vi "反应性主程序.vi"() -> ()   [LabVIEW 2020]
doc: "该范例演示了通过VI查看其它VI的方法，还可运行和中止查看的VI。\n对于要中止的VI，应设置为可中止。对于无法中止的VI，可查看相关范例。"
uses:
  <vilib>/Utility/error.llb/DialogType.ctl
  GlobalVariable.vi
  TCPModbus_MasterClient/MB Ethernet Master Query Write Multiple Registers (poly).vi
  TCPModbus_MasterClient/MB Ethernet Master Query Read Input Registers (poly).vi
  <vilib>/Analysis/polynomials.llb/Scalar Polynomial Evaluation (DBL).vi
  <vilib>/Analysis/NI_AALPro.lvlib
panel:
  out "上段":bool
  out "下段":bool
  in  "修正因子文件状态":bool
  out "退出":bool
  in  "Calculate Square":bool
  in  "Measure Square":bool
  in  "Physics Parameters Square":bool
  in  "Open Square":bool
  in  "Home Square":bool
  out "时间":string
  out "日期":string
  in  "MainPanel":enum32{"logo"}(tab)
  out "P2_8":dbl
  out "P2_7":dbl
  out "P2_6":dbl
  out "P2_5":dbl
  out "P2_4":dbl
  out "P2_3":dbl
  out "P2_2":dbl
  out "P2_1":dbl
  out "累计时差":dbl format="%#_2g"
  out "程序历时":dbl format="%#_2g"
  out "电脑历时":dbl format="%#_2g"
  out "脉冲3":dbl(knob) caption="Gauge" scale=1.0..1000000.0 scale format="%#_6p"
  out "脉冲2":dbl(knob) caption="Gauge" scale=1.0..1000000.0 scale format="%#_6p"
  out "电流 2":dbl(slide)=1.0 scale=1e-13..0.0001 scale format="%#_2e"
  out "电流 1":dbl(slide)=1.0 scale=1e-13..0.0001 scale format="%#_2e"
  out "电压8":dbl(knob) caption="Gauge" scale=1.0..5.0
  out "电压7":dbl(knob) caption="Gauge" scale=1.0..5.0
  out "电压6":dbl(knob) caption="Gauge" scale=1.0..5.0
  out "电压5":dbl(knob) caption="Gauge" scale=1.0..5.0
  out "电压4":dbl(knob) caption="Gauge" scale=1.0..5.0
  out "电压3":dbl(knob) caption="Gauge" scale=1.0..5.0
  out "电压2":dbl(knob) caption="Gauge" scale=1.0..5.0
  out "脉冲1":dbl(knob) caption="Gauge" scale=1.0..1000000.0 scale format="%#_6p"
  out "电压1":dbl(knob) caption="Gauge" scale=1.0..5.0
  in  "校准时间":bool
  in  "更新物理参数":bool
  in  "离线数据源":bool
  # "iRho-100型反应性仪"
  # "Network"
  # "Current1"
  # "Current2"
  # "Voltage Output"
  # "Voltage Input"
  # "AC220V/50Hz"
  # "Ground"
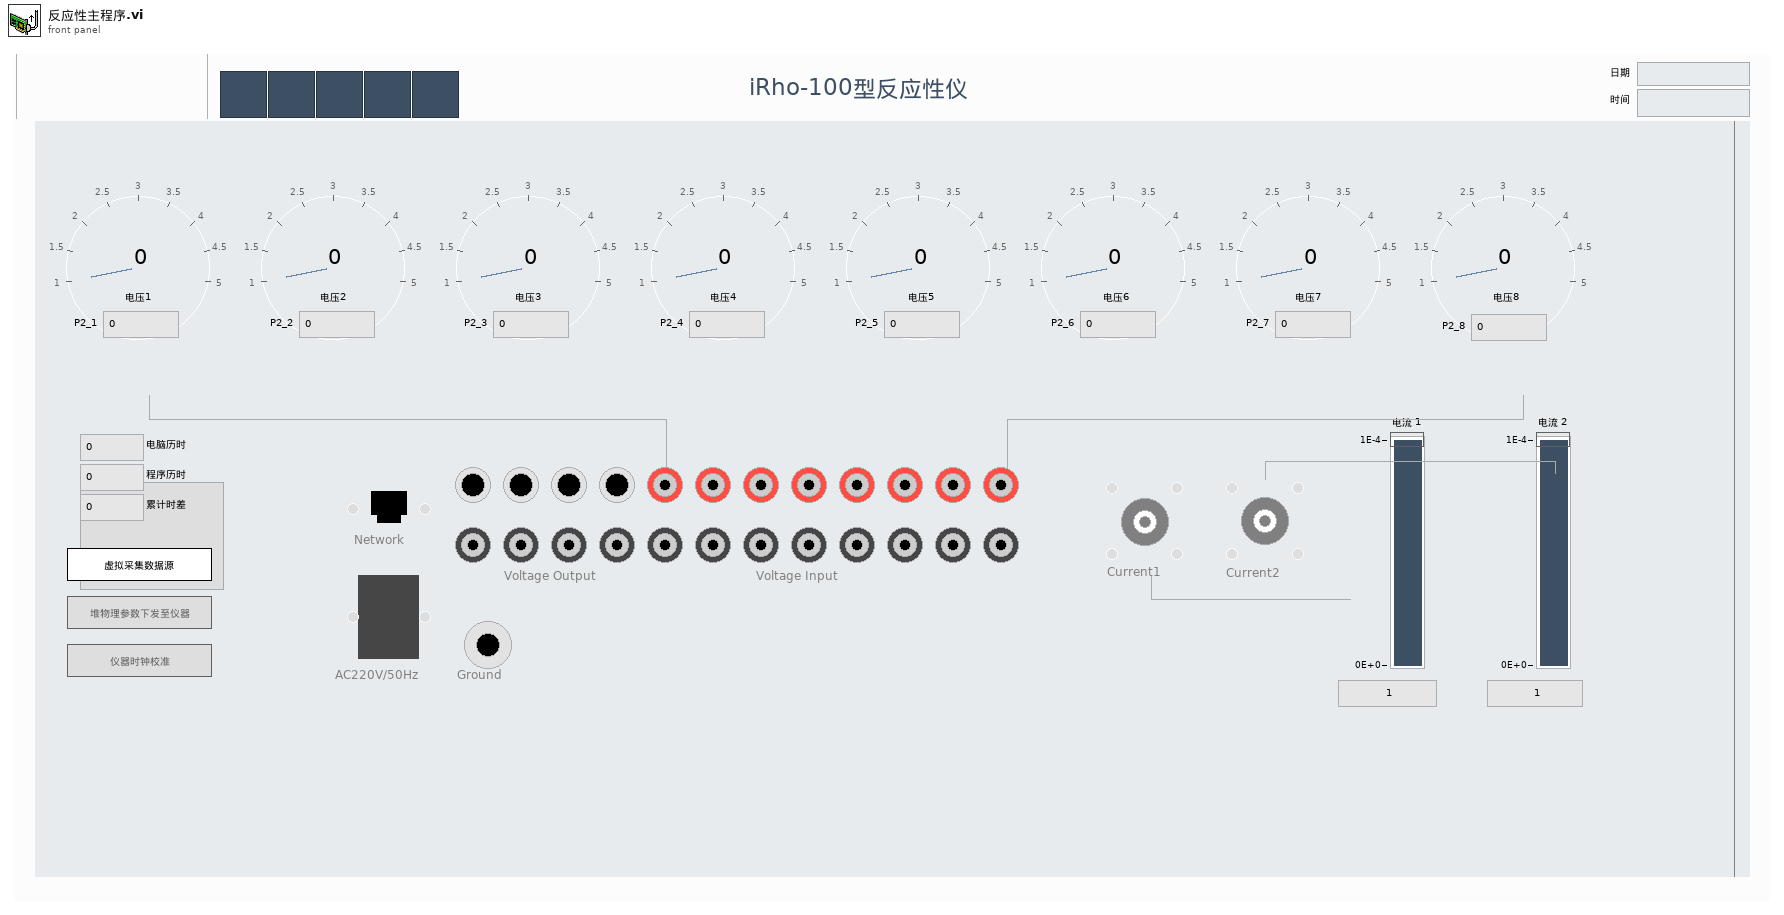
[diagram p1: front panel]
types:
  T1 = typedef "DialogType.ctl" = u16
  T2 = enum32{"Invalid", "Standard", "Closed", "Hidden", "Minimized", "Maximized"}
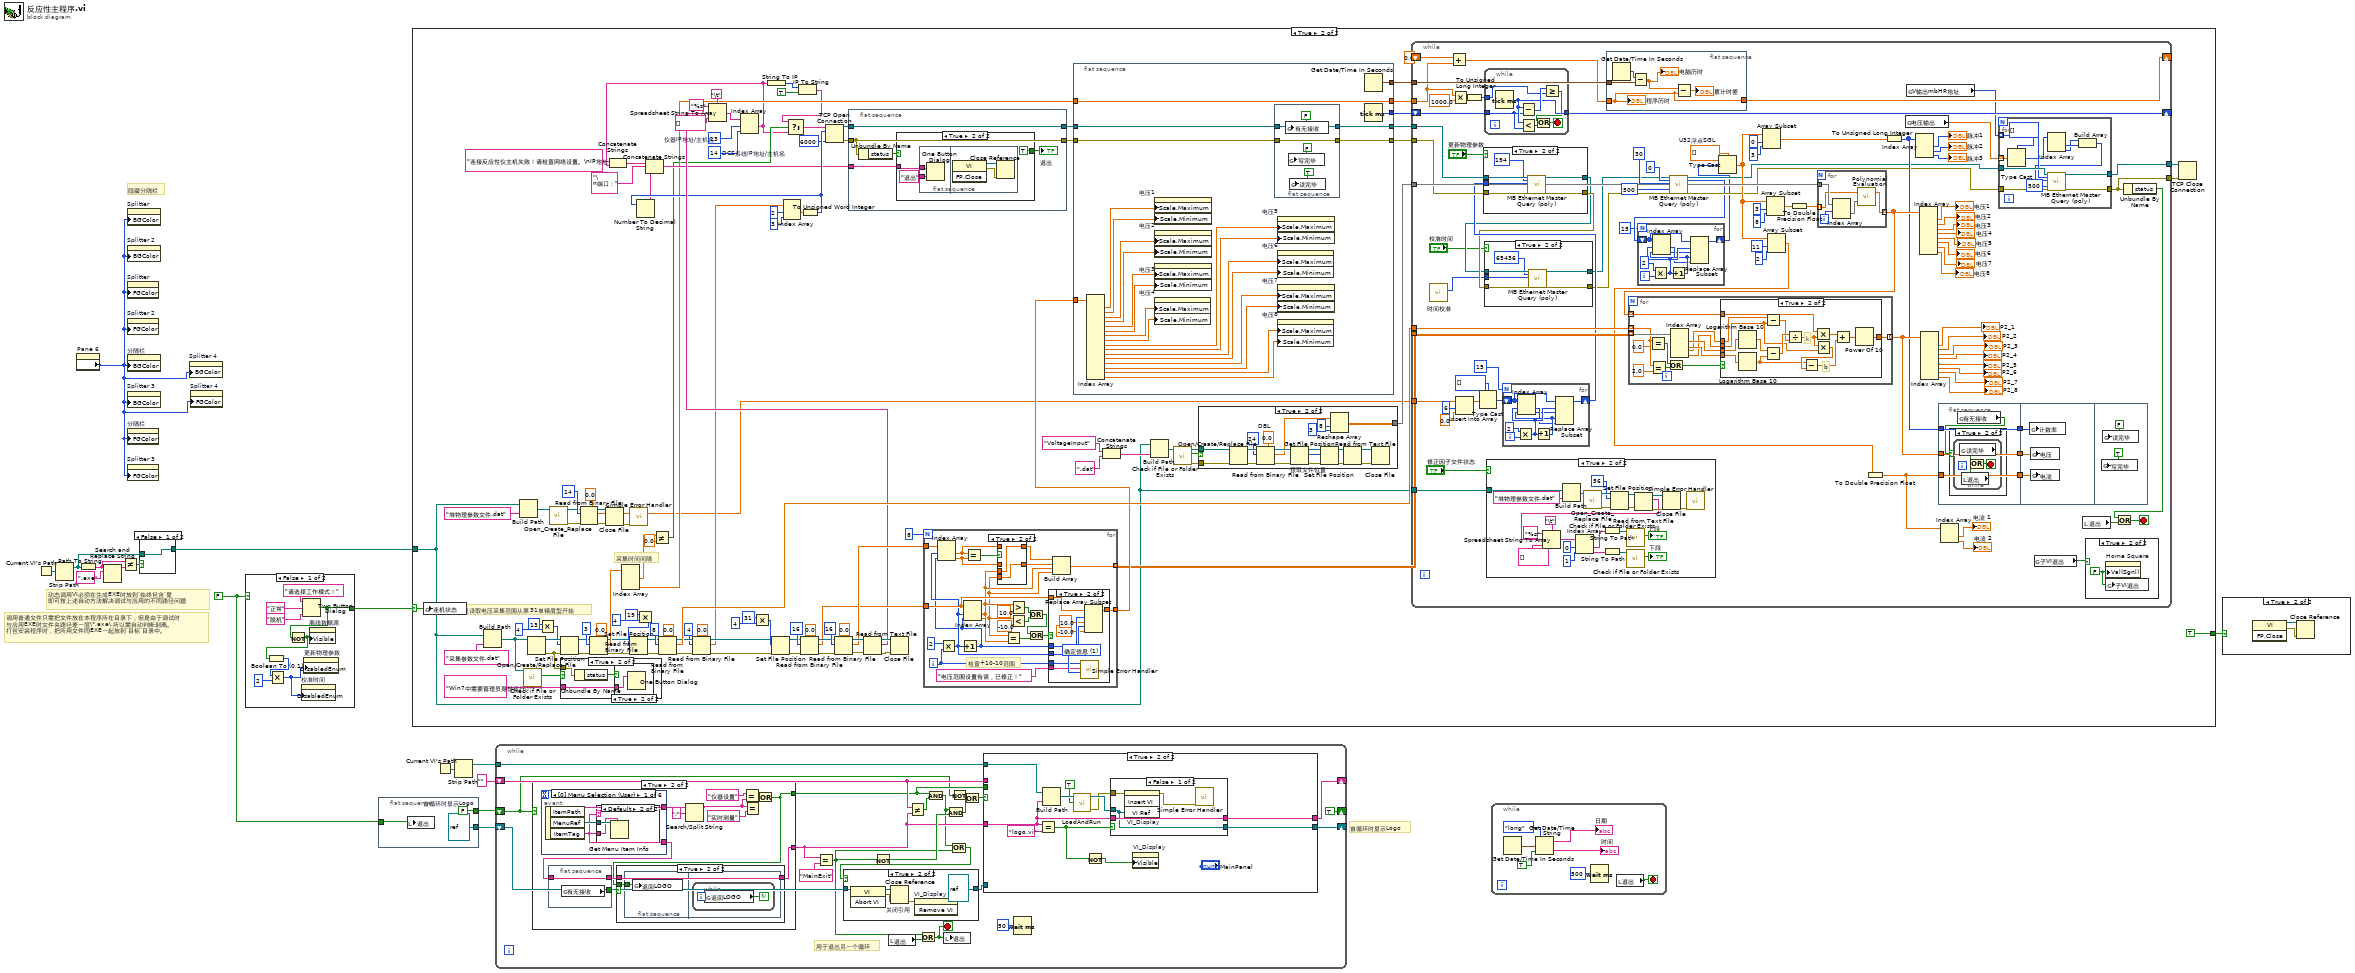
[diagram p0: block diagram]
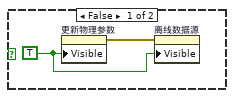
[diagram p2: hidden frame]
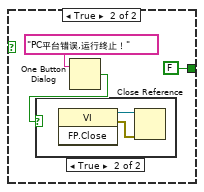
[diagram p3: hidden frame]
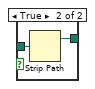
[diagram p5: hidden frame]
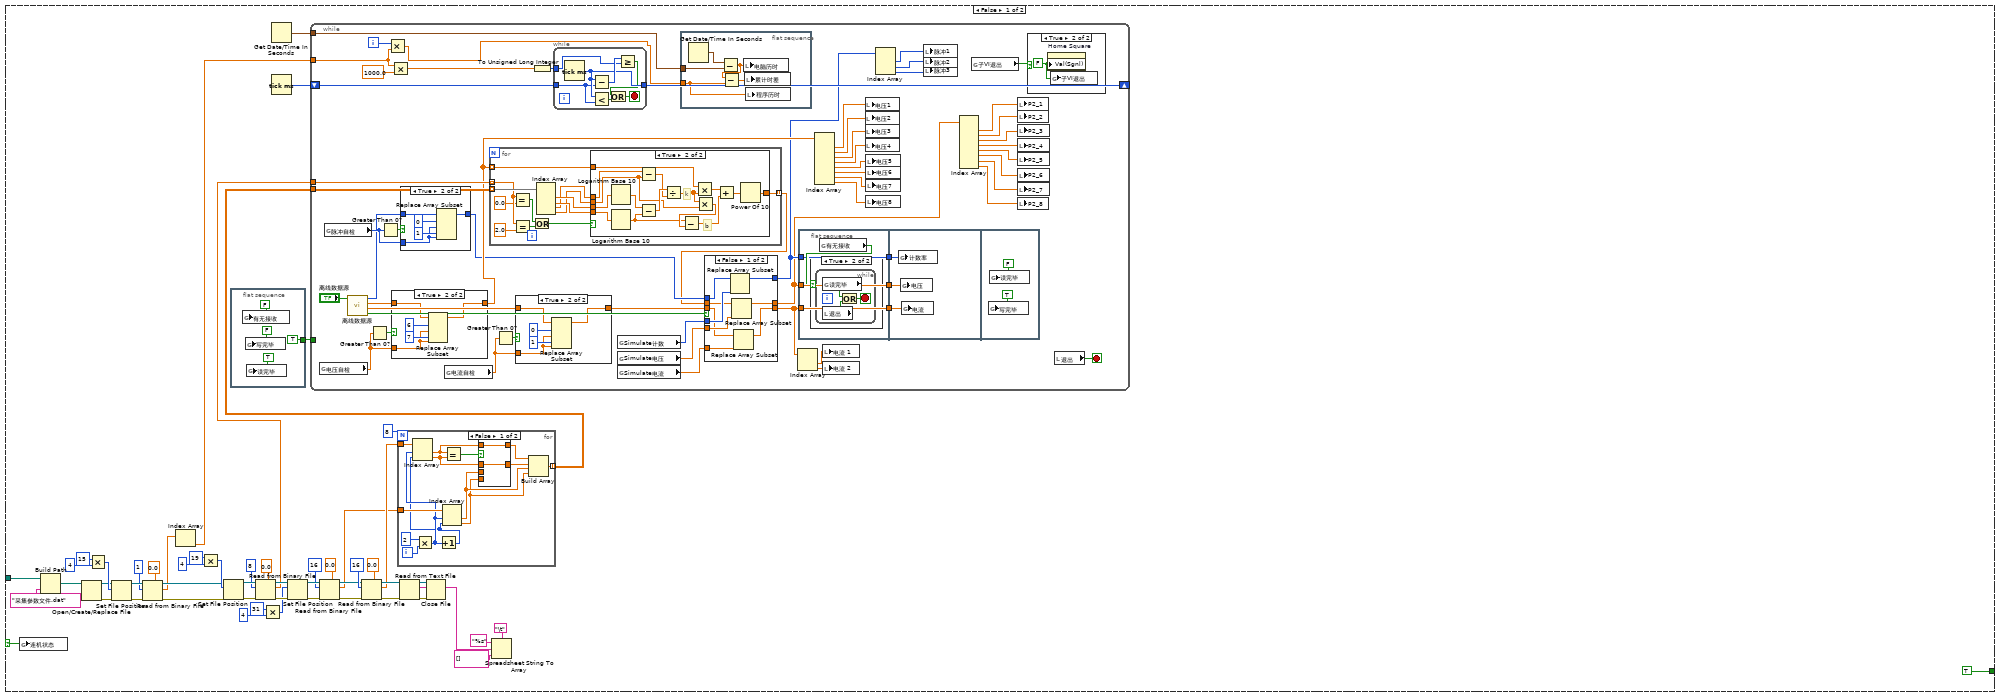
[diagram p6: hidden frame]
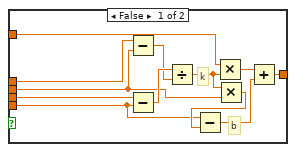
[diagram p12: hidden frame]
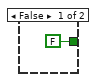
[diagram p15: hidden frame]
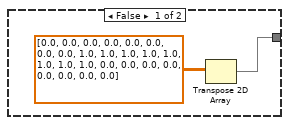
[diagram p18: hidden frame]
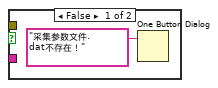
[diagram p19: hidden frame]
diagram:
  w2 = FALSE
  # "隐藏分隔栏"
  # "调用普通文件只需把文件放在本程序所在目录下，但是由于调试时\n与应用EXE时文件夹路径差一层\\*.exe\\,所以需自动判断剥离。\n打包安装程序时，把所用文件同EXE一起放到‘目标’目录中。"
  # "动态调用VI必须在生成EXE时放到‘始终包含’里\n即可按上述自动方法解决调试与应用的不同路径问题"
  # "首循环时显示Logo"
  n1 = Current VI's Path() -> (path=w11:path)
  n2 = Strip Path(path=w11) -> (stripped path=w6:path)  [unwired: 1 out]
  n3 = property on="Pane 6" class="Pane"() -> ("PaneColor"=w1:u32)  [unwired: 2 in, 2 out]
  n4 = Path To String(path=w6) -> (string=w8:string)
  n5 = Search and Replace String(input string=w8, search string=".exe" ("搜索字符串")) -> (result string=w9:string)  [unwired: 6 in, 3 out]
  n6 = Not Equal?(x=w8, y=w9) -> (x != y?=w7:bool)
  n7 = property on="Splitter" class="Splitter"("BGColor"=w1) -> ()  [unwired: 2 in, 2 out]
  n8 = property on="Splitter 2" class="Splitter"("BGColor"=w1) -> ()  [unwired: 2 in, 2 out]
  n9 = property on="Splitter" class="Splitter"("FGColor"=w1) -> ()  [unwired: 2 in, 2 out]
  n10 = property on="Splitter 2" class="Splitter"("FGColor"=w1) -> ()  [unwired: 2 in, 2 out]
  n11 = property on="分隔栏" class="Splitter"("BGColor"=w1) -> ()  [unwired: 2 in, 2 out]
  n12 = property on="Splitter 3" class="Splitter"("BGColor"=w1) -> ()  [unwired: 2 in, 2 out]
  n13 = property on="分隔栏" class="Splitter"("FGColor"=w1) -> ()  [unwired: 2 in, 2 out]
  n14 = property on="Splitter 3" class="Splitter"("FGColor"=w1) -> ()  [unwired: 2 in, 2 out]
  n15 = case shown="False" w7 {
    tunnel: w6 -> [w17 w19]
    tunnel: [w17 w18] -> w3
    frame False {
    }
    frame True {
      n16 = Strip Path(path=w19) -> (stripped path=w18:path)  [unwired: 1 out]
    }
  }
  n17 = property on="Splitter 4" class="Splitter"("BGColor"=w1) -> ()  [unwired: 2 in, 2 out]
  n18 = property on="Splitter 4" class="Splitter"("FGColor"=w1) -> ()  [unwired: 2 in, 2 out]
  n19 = case shown="False" w2 {
    tunnel: [w24 FALSE ("T button?")] -> w5
    frame False {
      n20 = Two Button Dialog(message="请选择工作模式！" ("消息"), 1:"脱机" ("F按钮名称（“取消”）"), 2:"正常" ("T按钮名称（“确定”）")) -> (T button?=w24:bool)
      n21 = Not(x=w24) -> (.not. x?=w23:bool)
      n22 = Boolean To (0,1)(Boolean=w23) -> (0, 1=w22:i16)
      n23 = Multiply(x=w22, y=i16 2) -> (x*y=w20:i16)
      n24 = property on="校准时间" class="Bool"("DisabledEnum"=w20) -> ()  [unwired: 2 in, 2 out]
      n25 = property on="更新物理参数" class="Bool"("DisabledEnum"=w20) -> ()  [unwired: 2 in, 2 out]
      n26 = property on="离线数据源" class="Bool"("Visible"=w23) -> ()  [unwired: 2 in, 2 out]
    }
    frame True {
      n27 = One Button Dialog(message="PC平台错误,运行终止！" ("消息")) -> (true=w28:bool)  [unwired: 1 in]
      n28 = case shown="True" w28 {
        frame False {
        }
        frame True {
          n29 = invoke class="VI" method="FP.Close"() -> (reference out=w31:refnum<vi>, error out=w32:errorcluster)  [unwired: 3 in, 1 out]
          n30 = Close Reference(reference=w31, error in (no error)=w32) -> ()  [unwired: 1 out]
        }
      }
    }
  }
  n31 = flat-sequence {
    tunnel: [refnum<vi> refnum ("VI Ref")] -> w16
    tunnel: [w34] -> w15
    tunnel: w2 -> [w33]
    frame #0 {
      w34 = FALSE  # 首循环时显示Logo
      n32 = local write "退出"(w33) -> ()
    }
  }
  n33 = case shown="True" w5 {
    selector: w5 -> [w38 w276]
    tunnel: w3 -> [w68 w270]
    tunnel: [TRUE ("首循环时显示Logo") TRUE ("首循环时显示Logo")] -> w4
    frame False {
      n34 = global write "GlobalVariable.vi" "连机状态"(w38) -> ()
      n35 = Build Path(base path=w68, name or relative path="采集参数文件.dat") -> (appended path=w70:path)
      n36 = Open/Create/Replace File(file path (use dialog)=w70) -> (refnum out=w58:refnum<file>, error out=w57:errorcluster)  [unwired: 5 in, 1 out]
      n37 = Multiply(x=i64 15 ("偏移量（字节）（0）"), y=i64 4 ("偏移量（字节）（0）")) -> (x*y=w65:i64)
      n38 = Set File Position(offset (in bytes) (0)=w65, refnum=w58, error in=w57) -> (refnum out=w61:refnum<file>, error out=w62:errorcluster)  [unwired: 1 in]
      n39 = Read from Binary File(5:sgl 0.0 ("byte stream type"), 8:w62, 10:1 ("count"), 11:w61) -> (0:w55:errorcluster, 2:w54:sgl[], 3:w56:refnum<file>)  [unwired: 2 in, 1 out]
      n40 = Index Array(array=w54) -> (element=w53:sgl)  [unwired: 1 in]
      n41 = Multiply(x=i64 19 ("偏移量（字节）（0）"), y=i64 4 ("偏移量（字节）（0）")) -> (x*y=w77:i64)
      n42 = Set File Position(offset (in bytes) (0)=w77, refnum=w56, error in=w55) -> (refnum out=w73:refnum<file>, error out=w74:errorcluster)  [unwired: 1 in]
      n43 = flat-sequence {
        tunnel: [TRUE ("读完毕")] -> w89
        frame #0 {
          n44 = global write "GlobalVariable.vi" "有无接收"(FALSE ("读完毕")) -> ()
          n45 = global write "GlobalVariable.vi" "写完毕"(FALSE ("读完毕")) -> ()
          n46 = global write "GlobalVariable.vi" "读完毕"(TRUE ("读完毕")) -> ()
        }
      }
      n47 = Read from Binary File(5:sgl 0.0 ("byte stream type"), 8:w74, 10:8 ("count"), 11:w73) -> (0:w85:errorcluster, 2:w67:sgl[], 3:w84:refnum<file>)  [unwired: 2 in, 1 out]
      n48 = Multiply(x=i64 31 ("偏移量（字节）（0）"), y=i64 4 ("偏移量（字节）（0）")) -> (x*y=w83:i64)
      n49 = Get Date/Time In Seconds() -> (seconds since 1Jan1904=w37:timestamp)
      n50 = Tick Count (ms)() -> (millisecond timer value=w36:u32)
      n51 = Set File Position(offset (in bytes) (0)=w83, refnum=w84, error in=w85) -> (refnum out=w80:refnum<file>, error out=w81:errorcluster)  [unwired: 1 in]
      n52 = Read from Binary File(5:sgl 0.0 ("byte stream type"), 8:w81, 10:16 ("count"), 11:w80) -> (0:w49:errorcluster, 2:w44:sgl[], 3:w50:refnum<file>)  [unwired: 2 in, 1 out]
      n53 = Read from Binary File(5:sgl 0.0 ("byte stream type"), 8:w49, 10:16 ("count"), 11:w50) -> (0:w47:errorcluster, 2:w45:sgl[], 3:w48:refnum<file>)  [unwired: 2 in, 1 out]
      n54 = for {
        N: 8 -> [_]
        tunnel: w44 -> [w102]
        tunnel: [w91] -> w43 mode=indexing
        tunnel: w45 -> [w90]
        i -> [w101]
        n55 = Multiply(x=2, y=w101) -> (x*y=w99:i32)
        n56 = Increment(x=w99) -> (x+1=w98:i32)
        n57 = Index Array(array=w90, index #1=w99, index #2=w98) -> (element #1=w97:sgl, element #2=w96:sgl)
        n58 = Index Array(array=w102, index #1=w99, index #2=w98) -> (element #1=w93:sgl, element #2=w92:sgl)
        n59 = Equal?(x=w97, y=w96) -> (x = y?=w100:bool)
        n60 = case shown="False" w100 {
          tunnel: w93 -> [_ w107]
          tunnel: w92 -> [_ w106]
          tunnel: [w105 w107] -> w95
          tunnel: w97 -> [w105 _]
          tunnel: w96 -> [w104 _]
          tunnel: [w104 w106] -> w94
          frame False {
          }
          frame True {
          }
        }
        n61 = Build Array(w95, w94, w93, w92) -> (w91:sgl[])
      }
      n62 = while {
        tunnel: w89 -> [_]
        tunnel: w67 -> [w162]
        tunnel: w53 -> [w139]
        tunnel: w43 -> [w163]
        tunnel: w37 -> [w135]
        shift-right: [w133] -> _
        shift-left: w36 -> [w136]
        i -> [w148]
        stop <- w166 stop-if-true
        n63 = global read "GlobalVariable.vi" "电压自检"() -> (w144:dbl)
        n64 = global read "GlobalVariable.vi" "脉冲自检"() -> (w142:i32)
        n65 = call "离线数据源.vi"("显示前面板"="离线数据源") -> ("前面板打开"=w129:bool, "电流"=w126:dbl[], "电压数据"=w127:dbl[], "脉冲数据"=w128:u32[])  [unwired: 7 in]
        n66 = Greater Than 0?(x=w144) -> (x > 0?=w145:bool)
        n67 = Greater Than 0?(x=w142) -> (x > 0?=w141:bool)
        n68 = Multiply(x=w148, y=w139) -> (x*y=w134:sgl)
        n69 = Multiply(x=w139, y=sgl 1000.0) -> (x*y=w137:sgl)
        n70 = case shown="True" w145 {
          tunnel: w127 -> [w200 w205]
          tunnel: [w200 w204] -> w143
          tunnel: w144 -> [_ w201]
          frame False {
          }
          frame True {
            n71 = Replace Array Subset(array=w205, new element #1=w201, index #1=6 ("索引"), new element #2=w201, index #2=7 ("索引")) -> (w204:dbl[])
          }
        }
        n72 = case shown="True" w141 {
          tunnel: w128 -> [w194 w199]
          tunnel: [w194 w198] -> w123
          tunnel: w142 -> [_ w195]
          frame False {
          }
          frame True {
            n73 = Replace Array Subset(array=w199, new element #1=w195, index #1=0 ("索引"), new element #2=w195, index #2=1 ("索引")) -> (w198:u32[])
          }
        }
        n74 = global read "GlobalVariable.vi" "电流自检"() -> (w146:dbl)
        n75 = for {
          tunnel: w143 -> [w223] mode=indexing
          tunnel: [w212] -> w119 mode=indexing
          tunnel: w163 -> [w224] mode=indexing
          tunnel: w162 -> [w222] mode=indexing
          n76 = Equal?(x=w222, y=sgl 0.0) -> (x = y?=w219:bool)
          n77 = Equal?(x=w222, y=sgl 2.0) -> (x = y?=w218:bool)
          n78 = Or(x=w219, y=w218) -> (x .or. y?=w217:bool)
          n79 = Index Array(array=w224) -> (element #1=w216:sgl, element #2=w215:sgl, element #3=w214:sgl, element #4=w213:sgl)  [unwired: 4 in]
          n80 = case shown="True" w217 {
            tunnel: w223 -> [w236 w242]
            tunnel: [w235 w240] -> w212
            tunnel: w214 -> [w228 w245]
            tunnel: w213 -> [w227 w244]
            tunnel: w216 -> [w226 w238]
            tunnel: w215 -> [w225 w243]
            frame False {
              # "b"
              # "k"
              n81 = Subtract(x=w228, y=w227) -> (x-y=w233:sgl)
              n82 = Subtract(x=w226, y=w225) -> (x-y=w234:sgl)
              n83 = Divide(x=w234, y=w233) -> (x/y=w232:sgl)
              n84 = Multiply(x=w236, y=w232) -> (x*y=w230:dbl)
              n85 = Multiply(x=w232, y=w227) -> (x*y=w231:sgl)
              n86 = Subtract(x=w225, y=w231) -> (x-y=w229:sgl)
              n87 = Add(x=w230, y=w229) -> (x+y=w235:dbl)
            }
            frame True {
              # "b"
              # "k"
              n88 = Logarithm Base 10(1:w238) -> (0:w237:sgl)
              n89 = Logarithm Base 10(1:w243) -> (0:w239:sgl)
              n90 = Subtract(x=w245, y=w244) -> (x-y=w250:sgl)
              n91 = Subtract(x=w237, y=w239) -> (x-y=w251:sgl)
              n92 = Divide(x=w251, y=w250) -> (x/y=w249:sgl)
              n93 = Multiply(x=w242, y=w249) -> (x*y=w247:dbl)
              n94 = Multiply(x=w249, y=w244) -> (x*y=w248:sgl)
              n95 = Subtract(x=w239, y=w248) -> (x-y=w246:sgl)
              n96 = Add(x=w247, y=w246) -> (x+y=w241:dbl)
              n97 = Power Of 10(x=w241) -> (10^x=w240:dbl)
            }
          }
        }
        n98 = Greater Than 0?(x=w146) -> (x > 0?=w147:bool)
        n99 = case shown="True" w147 {
          tunnel: w126 -> [w206 w211]
          tunnel: [w206 w210] -> w125
          tunnel: w146 -> [_ w207]
          frame False {
          }
          frame True {
            n100 = Replace Array Subset(array=w211, new element #1=w207, index #1=0 ("索引"), new element #2=w207, index #2=1 ("索引")) -> (w210:dbl[])
          }
        }
        n101 = To Unsigned Long Integer(number=w137) -> (unsigned 32bit integer=w140:u32)
        n102 = while {
          tunnel: w136 -> [w190]
          tunnel: w140 -> [w192]
          tunnel: [w191] -> w133
          stop <- w187 stop-if-true
          n103 = Tick Count (ms)() -> (millisecond timer value=w191:u32)
          n104 = Subtract(x=w191, y=w190) -> (x-y=w193:u32)
          n105 = Less?(x=w191, y=w190) -> (x < y?=w189:bool)
          n106 = Greater Or Equal?(x=w193, y=w192) -> (x >= y?=w188:bool)
          n107 = Or(x=w188, y=w189) -> (x .or. y?=w187:bool)
        }
        n108 = global read "GlobalVariable.vi" "Simulate计数"() -> (w132:u32[])
        n109 = global read "GlobalVariable.vi" "Simulate电压"() -> (w131:dbl[])
        n110 = global read "GlobalVariable.vi" "Simulate电流"() -> (w130:dbl[])
        n111 = flat-sequence {
          tunnel: w135 -> [w185]
          tunnel: w134 -> [w182]
          frame #0 {
            n112 = Get Date/Time In Seconds() -> (seconds since 1Jan1904=w186:timestamp)
            n113 = Subtract(x=w186, y=w185) -> (x-y=w183:dbl)
            n114 = Subtract(x=w183, y=w182) -> (x-y=w184:dbl)
            n115 = local write "电脑历时"(w183) -> ()
            n116 = local write "累计时差"(w184) -> ()
            n117 = local write "程序历时"(w182) -> ()
          }
        }
        n118 = case shown="False" w129 {
          tunnel: w123 -> [w178 w181]
          tunnel: w119 -> [w174 w180]
          tunnel: w125 -> [w170 w179]
          tunnel: [w176 w181] -> w122
          tunnel: [w173 w180] -> w112
          tunnel: [w172 w179] -> w124
          tunnel: w132 -> [w177 _]
          tunnel: w131 -> [w175 _]
          tunnel: w130 -> [w171 _]
          frame False {
            n119 = Replace Array Subset(array=w178, new element=w177) -> (w176:u32[])  [unwired: 1 in]
            n120 = Replace Array Subset(array=w174, new element=w175) -> (w173:dbl[])  [unwired: 1 in]
            n121 = Replace Array Subset(array=w170, new element=w171) -> (w172:dbl[])  [unwired: 1 in]
          }
          frame True {
          }
        }
        n122 = Index Array(array=w124) -> (element #1=w161:dbl, element #2=w160:dbl)  [unwired: 2 in]
        n123 = flat-sequence {
          tunnel: w124 -> [w255]
          tunnel: w112 -> [w256]
          tunnel: [w256] -> w169
          tunnel: [w255] -> w168
          tunnel: [w253] -> w167
          tunnel: w122 -> [w253]
          tunnel: w169 -> [w262]
          tunnel: w168 -> [w261]
          tunnel: w167 -> [w260]
          frame #0 {
            n124 = global read "GlobalVariable.vi" "有无接收"() -> (w254:bool)
            n125 = case shown="True" w254 {
              frame False {
              }
              frame True {
                n126 = while {
                  stop <- w259 stop-if-true
                  n127 = global read "GlobalVariable.vi" "读完毕"() -> (w258:bool)
                  n128 = local read "退出"() -> (w257:bool)
                  n129 = Or(x=w258, y=w257) -> (x .or. y?=w259:bool)
                }
              }
            }
          }
          frame #1 {
            n130 = global write "GlobalVariable.vi" "计数率"(w260) -> ()
            n131 = global write "GlobalVariable.vi" "电压"(w262) -> ()
            n132 = global write "GlobalVariable.vi" "电流"(w261) -> ()
          }
          frame #2 {
            n133 = global write "GlobalVariable.vi" "写完毕"(TRUE ("写完毕")) -> ()
            n134 = global write "GlobalVariable.vi" "读完毕"(FALSE ("写完毕")) -> ()
          }
        }
        n135 = Index Array(array=w143) -> (element #1=w156:dbl, element #2=w155:dbl, element #3=w154:dbl, element #4=w153:dbl, element #5=w152:dbl, element #6=w151:dbl, element #7=w150:dbl, element #8=w149:dbl)  [unwired: 8 in]
        n136 = local write "电流 1"(w161) -> ()
        n137 = local write "电流 2"(w160) -> ()
        n138 = local write "电压1"(w156) -> ()
        n139 = local write "电压2"(w155) -> ()
        n140 = local write "电压3"(w154) -> ()
        n141 = local write "电压4"(w153) -> ()
        n142 = local write "电压5"(w152) -> ()
        n143 = local write "电压6"(w151) -> ()
        n144 = local write "电压7"(w150) -> ()
        n145 = local write "电压8"(w149) -> ()
        n146 = Index Array(array=w122) -> (element #1=w159:u32, element #2=w158:u32, element #3=w157:u32)  [unwired: 3 in]
        n147 = local write "脉冲1"(w159) -> ()
        n148 = local write "脉冲2"(w158) -> ()
        n149 = local write "脉冲3"(w157) -> ()
        n150 = Index Array(array=w112) -> (element #1=w121:dbl, element #2=w120:dbl, element #3=w118:dbl, element #4=w117:dbl, element #5=w116:dbl, element #6=w115:dbl, element #7=w114:dbl, element #8=w113:dbl)  [unwired: 8 in]
        n151 = global read "GlobalVariable.vi" "子VI退出"() -> (w164:bool)
        n152 = local write "P2_1"(w121) -> ()
        n153 = local write "P2_2"(w120) -> ()
        n154 = local write "P2_8"(w113) -> ()
        n155 = local write "P2_3"(w118) -> ()
        n156 = local write "P2_4"(w117) -> ()
        n157 = local write "P2_5"(w116) -> ()
        n158 = local write "P2_6"(w115) -> ()
        n159 = local write "P2_7"(w114) -> ()
        n160 = case shown="True" w164 {
          frame False {
          }
          frame True {
            w252 = FALSE ("值(信号)")
            n161 = property on="Home Square" class="Bool (strict)"("Val(Sgnl)"=w252) -> ()  [unwired: 2 in, 2 out]
            n162 = global write "GlobalVariable.vi" "子VI退出"(w252) -> ()
          }
        }
        n163 = local read "退出"() -> (w166:bool)
      }
      n164 = Read from Text File(file (use dialog)=w48, error in=w47) -> (refnum out=w87:refnum<file>, text=w39:string, error out=w86:errorcluster)  [unwired: 1 in, 2 out]
      n165 = Close File(refnum=w87, error in=w86) -> ()  [unwired: 2 out]
      n166 = Spreadsheet String To Array(delimiter (Tab)="\t", format string="%s", spreadsheet string=w39, array type (2D Dbl)=string[] [] ("添加的数组")) -> ()  [unwired: 1 out]
    }
    frame True {
      w303 = 14  # DCS系统IP地址/主机名
      w304 = 13  # 仪器IP地址/主机名
      # "采集时间间隔"
      # "只读取电压采集范围从第31单精度型开始"
      n167 = global write "GlobalVariable.vi" "连机状态"(w276) -> ()
      n168 = Build Path(base path=w270, name or relative path="采集参数文件.dat") -> (appended path=w351:path)
      n169 = Build Path(base path=w270, name or relative path="堆物理参数文件.dat" ("string")) -> (appended path=w272:path)
      n170 = call <vilib>:"Check if File or Folder Exists.vi"("path"=w351) -> ("file or folder exists?"=w350:bool)  [unwired: 8 in, 2 out]
      n171 = Open/Create/Replace File(file path (use dialog)=w351) -> (refnum out=w359:refnum<file>, error out=w349:errorcluster)  [unwired: 5 in, 1 out]
      n172 = Multiply(x=i64 13 ("偏移量（字节）（0）"), y=i64 4 ("偏移量（字节）（0）")) -> (x*y=w356:i64)
      n173 = call <vilib>:"Open_Create_Replace File.vi"("file path"=w272) -> ("error out"=w266:errorcluster, "refnum"=w267:refnum<file>)  [unwired: 7 in, 2 out]
      n174 = Set File Position(offset (in bytes) (0)=w356, refnum=w359, error in=w349) -> (refnum out=w361:refnum<file>, error out=w360:errorcluster)  [unwired: 1 in]
      n175 = case shown="True" w350 {
        tunnel: w349 -> [_ w449]
        tunnel: "Win7中需要管理员身份运行！" -> [_ w447]
        frame False {
          n176 = One Button Dialog(message="采集参数文件.dat不存在！" ("消息")) -> ()  [unwired: 1 in, 1 out]
        }
        frame True {
          n177 = Unbundle By Name(w449) -> ("status"=w448:bool)
          n178 = case shown="True" w448 {
            tunnel: w447 -> [_ w450]
            frame False {
            }
            frame True {
              n179 = One Button Dialog(message=w450) -> ()  [unwired: 1 in, 1 out]
            }
          }
        }
      }
      n180 = Read from Binary File(5:sgl 0.0, 8:w266, 10:14, 11:w267) -> (0:w268:errorcluster, 2:w265:sgl[], 3:w269:refnum<file>)  [unwired: 2 in, 1 out]
      n181 = Read from Binary File(5:sgl 0.0 ("byte stream type"), 8:w360, 10:3 ("count"), 11:w361) -> (0:w342:errorcluster, 2:w354:sgl[], 3:w343:refnum<file>)  [unwired: 2 in, 1 out]
      n182 = Close File(refnum=w269, error in=w268) -> (error out=w271:errorcluster)  [unwired: 1 out]
      n183 = Index Array(array=w354) -> (element #1=w284:sgl, element #3=w286:sgl)  [unwired: 3 in, 1 out]
      n184 = call <vilib>:"Simple Error Handler.vi"("error in (no error)"=w271) -> ()  [unwired: 4 in, 5 out]
      n185 = Multiply(x=i64 19 ("偏移量（字节）（0）"), y=i64 4 ("偏移量（字节）（0）")) -> (x*y=w339:i64)
      n186 = Set File Position(offset (in bytes) (0)=w339, refnum=w343, error in=w342) -> (refnum out=w345:refnum<file>, error out=w344:errorcluster)  [unwired: 1 in]
      n187 = Not Equal?(x=w284, y=sgl 0.0) -> (x != y?=w282:bool)
      n188 = Read from Binary File(5:sgl 0.0 ("byte stream type"), 8:w344, 10:8 ("count"), 11:w345) -> (0:w301:errorcluster, 2:w338:sgl[], 3:w300:refnum<file>)  [unwired: 2 in, 1 out]
      n189 = Read from Binary File(5:sgl 0.0 ("byte stream type"), 8:w301, 10:4 ("count"), 11:w300) -> (0:w298:errorcluster, 2:w296:sgl[], 3:w299:refnum<file>)  [unwired: 2 in, 1 out]
      n190 = Multiply(x=i64 31 ("偏移量（字节）（0）"), y=i64 4 ("偏移量（字节）（0）")) -> (x*y=w364:i64)
      n191 = Set File Position(offset (in bytes) (0)=w364, refnum=w299, error in=w298) -> (refnum out=w370:refnum<file>, error out=w369:errorcluster)  [unwired: 1 in]
      n192 = Index Array(array=w296, index #1=2 ("索引"), index #2=3 ("索引")) -> (element #1=w295:sgl)  [unwired: 1 out]
      n193 = Read from Binary File(5:sgl 0.0 ("byte stream type"), 8:w369, 10:16 ("count"), 11:w370) -> (0:w328:errorcluster, 2:w324:sgl[], 3:w329:refnum<file>)  [unwired: 2 in, 1 out]
      n194 = To Unsigned Word Integer(number=w295) -> (unsigned 16bit integer=w292:u16)
      n195 = Number To Decimal String(number=w292) -> (decimal integer string=w291:string)  [unwired: 1 in]
      n196 = Read from Binary File(5:sgl 0.0 ("byte stream type"), 8:w328, 10:16 ("count"), 11:w329) -> (0:w326:errorcluster, 2:w325:sgl[], 3:w327:refnum<file>)  [unwired: 2 in, 1 out]
      n197 = flat-sequence {
        tunnel: w315 -> [w379]
        tunnel: w314 -> [w378]
        tunnel: [w379] -> w313
        tunnel: [w378] -> w312
        tunnel: w289 -> [w375]
        frame #0 {
          n198 = Unbundle By Name(w378) -> ("status"=w377:bool)
          n199 = case shown="True" w377 {
            tunnel: [FALSE ("退出") TRUE ("退出")] -> w376
            tunnel: w375 -> [_ w382]
            frame False {
            }
            frame True {
              n200 = flat-sequence {
                tunnel: w382 -> [w385]
                tunnel: "退出" ("按钮名称（“确定”）") -> [w384]
                frame #0 {
                  n201 = One Button Dialog(message=w385, button name ("OK")=w384) -> ()  [unwired: 1 out]
                }
                frame #1 {
                  n202 = invoke class="VI" method="FP.Close"() -> (reference out=w386:refnum<vi>, error out=w387:errorcluster)  [unwired: 3 in, 1 out]
                  n203 = Close Reference(reference=w386, error in (no error)=w387) -> ()  [unwired: 1 out]
                }
              }
            }
          }
          "退出" <- w376
        }
      }
      n204 = Read from Text File(file (use dialog)=w327, error in=w326) -> (refnum out=w367:refnum<file>, text=w306:string, error out=w368:errorcluster)  [unwired: 1 in, 2 out]
      n205 = Spreadsheet String To Array(delimiter (Tab)="\t", format string="%s", spreadsheet string=w306, array type (2D Dbl)=string[] [] ("添加的数组")) -> (array=w305:string[])
      n206 = Index Array(array=w305, index #1=w304, index #2=w303) -> (element #1=w281:string)  [unwired: 1 out]
      n207 = Concatenate Strings("连接反应性仪主机失败！请检查网络设置。\nIP地址：" ("消息"), w281) -> (w293:string)
      n208 = Concatenate Strings(w293, "\n端口：" ("字符串"), w291) -> (w289:string)
      n209 = String To IP(1:w281) -> (0:w279:u32)
      n210 = IP To String(1:TRUE ("句点符号？(F)"), 2:w279) -> (0:w278:string)
      n211 = Select(t=w278, s=w282, f=w281) -> (s? t:f=w283:string)
      n212 = TCP Open Connection(address=w283, remote port or service name=w292, timeout ms (60000)=6000 ("超时毫秒(60000)")) -> (connection ID=w315:refnum<k5>, error out=w314:errorcluster)  [unwired: 1 in, 1 out]
      n213 = Close File(refnum=w367, error in=w368) -> ()  [unwired: 2 out]
      n214 = for {
        N: 8 -> [_]
        tunnel: w324 -> [w405]
        tunnel: [w404] -> w323
        tunnel: [w389] -> w322 mode=indexing
        tunnel: w325 -> [w388]
        i -> [w402]
        # "检查+10-10范围"
        n215 = Multiply(x=2, y=w402) -> (x*y=w400:i32)
        n216 = Increment(x=w400) -> (x+1=w399:i32)
        n217 = Index Array(array=w388, index #1=w400, index #2=w399) -> (element #1=w398:sgl, element #2=w397:sgl)
        n218 = Index Array(array=w405, index #1=w400, index #2=w399) -> (element #1=w391:sgl, element #2=w390:sgl)
        n219 = Equal?(x=w398, y=w397) -> (x = y?=w401:bool)
        n220 = case shown="True" w401 {
          tunnel: w391 -> [_ w414]
          tunnel: w390 -> [_ w413]
          tunnel: [w412 w414] -> w393
          tunnel: w398 -> [w412 _]
          tunnel: w397 -> [w411 _]
          tunnel: [w411 w413] -> w392
          frame False {
          }
          frame True {
          }
        }
        n221 = Equal?(x=w390, y=w391) -> (x = y?=w395:bool)
        n222 = Greater?(x=w391, y=10.0) -> (0:w407:bool)
        n223 = Less?(x=w390, y=sgl -10.0) -> (x < y?=w406:bool)
        n224 = Or(x=w407, y=w406) -> (x .or. y?=w396:bool)
        n225 = Or(x=w396, y=w395) -> (x .or. y?=w394:bool)
        n226 = case shown="True" w394 {
          tunnel: w405 -> [w415 w424]
          tunnel: [w415 w423] -> w404
          tunnel: w399 -> [_ w422]
          tunnel: w400 -> [_ w421]
          tunnel: "电压范围设置有误，已修正！" ("error source (\" \")") -> [_ w417]
          tunnel: w402 -> [_ w416]
          frame False {
          }
          frame True {
            w418 = T1 1 items=["无对话框", "确定信息", "继续或停止信息", "确定信息＋警告", "继续/停止+警告"] ("type of dialog (OK msg:1)")
            n227 = call <vilib>:"Simple Error Handler.vi"("error code (no error:0)"=w416, "error source (\" \")"=w417, "type of dialog (OK msg:1)"=w418) -> ()  [unwired: 2 in, 5 out]
            n228 = Replace Array Subset(array=w424, new element #1=sgl 10.0 ("新元素/子数组"), index #1=w421, new element #2=sgl -10.0 ("新元素/子数组"), index #2=w422) -> (w423:sgl[])
          }
        }
        n229 = Build Array(w393, w392, w391, w390) -> (w389:sgl[])
      }
      n230 = flat-sequence {
        tunnel: [w474] -> w374
        tunnel: w323 -> [w473]
        tunnel: [w456] -> w363
        tunnel: w286 -> [w456]
        tunnel: [w451] -> w319
        tunnel: [w453] -> w318
        tunnel: [w455] -> w317
        tunnel: w313 -> [w452]
        tunnel: w312 -> [w454]
        frame #0 {
          n231 = Index Array(array=w473) -> (element #1=w465:sgl, element #2=w472:sgl, element #3=w464:sgl, element #4=w463:sgl, element #5=w462:sgl, element #6=w471:sgl, element #7=w461:sgl, element #8=w470:sgl, element #9=w460:sgl, element #10=w469:sgl, element #11=w459:sgl, element #12=w468:sgl, element #13=w458:sgl, element #14=w467:sgl, element #15=w457:sgl, element #16=w466:sgl)  [unwired: 16 in]
          n232 = property on="电压4" class="Knob (strict)"("Scale.Maximum"=w461, "Scale.Minimum"=w470) -> ()  [unwired: 2 in, 2 out]
          n233 = property on="电压1" class="Knob (strict)"("Scale.Maximum"=w465, "Scale.Minimum"=w472) -> ()  [unwired: 2 in, 2 out]
          n234 = property on="电压2" class="Knob (strict)"("Scale.Maximum"=w464, "Scale.Minimum"=w463) -> ()  [unwired: 2 in, 2 out]
          n235 = property on="电压3" class="Knob (strict)"("Scale.Maximum"=w462, "Scale.Minimum"=w471) -> ()  [unwired: 2 in, 2 out]
          n236 = flat-sequence {
            tunnel: w454 -> [w476]
            tunnel: [w476] -> w453
            tunnel: w452 -> [w475]
            tunnel: [w475] -> w451
            frame #0 {
              n237 = global write "GlobalVariable.vi" "有无接收"(FALSE ("读完毕")) -> ()
              n238 = global write "GlobalVariable.vi" "写完毕"(FALSE ("读完毕")) -> ()
              n239 = global write "GlobalVariable.vi" "读完毕"(TRUE ("读完毕")) -> ()
            }
          }
          n240 = property on="电压6" class="Knob (strict)"("Scale.Maximum"=w459, "Scale.Minimum"=w468) -> ()  [unwired: 2 in, 2 out]
          n241 = property on="电压8" class="Knob (strict)"("Scale.Maximum"=w457, "Scale.Minimum"=w466) -> ()  [unwired: 2 in, 2 out]
          n242 = property on="电压5" class="Knob (strict)"("Scale.Maximum"=w460, "Scale.Minimum"=w469) -> ()  [unwired: 2 in, 2 out]
          n243 = property on="电压7" class="Knob (strict)"("Scale.Maximum"=w458, "Scale.Minimum"=w467) -> ()  [unwired: 2 in, 2 out]
          n244 = Get Date/Time In Seconds() -> (seconds since 1Jan1904=w474:timestamp)
          n245 = Tick Count (ms)() -> (millisecond timer value=w455:u32)
        }
      }
      n246 = Concatenate Strings("VoltageInput", ".dat") -> (w332:string)
      n247 = Build Path(base path=w270, name or relative path=w332) -> (appended path=w337:path)
      n248 = call <vilib>:"Check if File or Folder Exists.vi"("path"=w337) -> ("error out"=w335:errorcluster, "file or folder exists?"=w334:bool, "dup path"=w336:path)  [unwired: 8 in]
      n249 = case shown="True" w334 {
        tunnel: [w425 w429] -> w352
        tunnel: w336 -> [_ w428]
        tunnel: w335 -> [_ w427]
        frame False {
          n250 = Transpose 2D Array(2D array=dbl[][] [[0.0, 0.0, 0.0, 0.0, 0.0, 0.0, 0.0, 0.0], [1.0, 1.0, 1.0, 1.0, 1.0, 1.0, 1.0, 1.0], [0.0, 0.0, 0.0, 0.0, 0.0, 0.0, 0.0, 0.0]]) -> (transposed array=w425:dbl[][])
        }
        frame True {
          w442 = 0.0  # DBL
          n251 = Open/Create/Replace File(file path (use dialog)=w428, error in=w427) -> (refnum out=w445:refnum<file>, error out=w444:errorcluster)  [unwired: 4 in, 1 out]
          n252 = Read from Binary File(5:w442, 8:w444, 10:24 ("count"), 11:w445) -> (0:w433:errorcluster, 2:w430:dbl[], 3:w434:refnum<file>)  [unwired: 2 in, 1 out]
          n253 = Get File Position "获取文件位置"(4:w433, 7:w434) -> (0:w440:errorcluster, 2:w439:i64, 3:w441:refnum<file>)
          n254 = Set File Position(offset (in bytes) (0)=w439, refnum=w441, error in=w440) -> (refnum out=w438:refnum<file>, error out=w437:errorcluster)  [unwired: 1 in]
          n255 = Reshape Array(w430, 8 ("维数大小"), 3 ("维数大小")) -> (w429:dbl[][])
          n256 = Read from Text File(file (use dialog)=w438, error in=w437) -> (refnum out=w436:refnum<file>, error out=w435:errorcluster)  [unwired: 1 in, 3 out]
          n257 = Close File(refnum=w436, error in=w435) -> ()  [unwired: 2 out]
        }
      }
      n258 = while {
        tunnel: w363 -> [w538]
        tunnel: w374 -> [w564]
        tunnel: w352 -> [w563]
        tunnel: w338 -> [w561]
        tunnel: w322 -> [w560]
        tunnel: w319 -> [w524]
        tunnel: w318 -> [w523]
        shift-right: [w540] -> _
        shift-left: w317 -> [w544]
        shift-right: [w536] -> _
        shift-left: sgl 0.0 ("byte stream type") -> [w539]
        tunnel: [w529] -> w311
        tunnel: [w530] -> w310
        tunnel: w270 -> [w526]
        tunnel: w265 -> [w515]
        stop <- w535 stop-if-true
        w512 = sgl[] []  # U32浮点SGL
        n259 = call "时间校准.vi"() -> ("DTout"=w502:u16[])  [unwired: 11 in]
        n260 = Add(x=w539, y=w538) -> (x+y=w537:sgl)
        n261 = Multiply(x=w538, y=sgl 1000.0) -> (x*y=w542:sgl)
        n262 = Insert Into Array(array=w515, index=6 ("索引"), new element=sgl 0.0 ("新元素/子数组")) -> (w516:sgl[])
        n263 = To Unsigned Long Integer(number=w542) -> (unsigned 32bit integer=w541:u32)
        n264 = Type Cast(type=u16[] [] ("Input Registers"), x=w516) -> (*(type *) &x=w520:u16[])
        n265 = while {
          tunnel: w544 -> [w639]
          tunnel: w541 -> [w641]
          tunnel: [w640] -> w540
          stop <- w636 stop-if-true
          n266 = Tick Count (ms)() -> (millisecond timer value=w640:u32)
          n267 = Subtract(x=w640, y=w639) -> (x-y=w642:u32)
          n268 = Less?(x=w640, y=w639) -> (x < y?=w638:bool)
          n269 = Greater Or Equal?(x=w642, y=w641) -> (x >= y?=w637:bool)
          n270 = Or(x=w637, y=w638) -> (x .or. y?=w636:bool)
        }
        n271 = case shown="True" "修正因子文件状态" {
          tunnel: w526 -> [_ w604]
          frame False {
          }
          frame True {
            n272 = Build Path(base path=w604, name or relative path="堆物理参数文件.dat" ("string")) -> (appended path=w622:path)
            n273 = call <vilib>:"Open_Create_Replace File.vi"("file path"=w622) -> ("error out"=w620:errorcluster, "refnum"=w621:refnum<file>)  [unwired: 7 in, 2 out]
            n274 = Set File Position(offset (in bytes) (0)=i64 56 ("偏移量（字节）（0）"), refnum=w621, error in=w620) -> (refnum out=w610:refnum<file>, error out=w609:errorcluster)  [unwired: 1 in]
            n275 = Read from Text File(file (use dialog)=w610, error in=w609) -> (refnum out=w607:refnum<file>, text=w605:string, error out=w606:errorcluster)  [unwired: 1 in, 2 out]
            n276 = Spreadsheet String To Array(delimiter (Tab)="\t", format string="%s", spreadsheet string=w605, array type (2D Dbl)=string[] [] ("添加的数组")) -> (array=w613:string[])
            n277 = Index Array(array=w613, index #1=0 ("index"), index #2=1 ("index")) -> (element #1=w612:string, element #2=w602:string)
            n278 = String To Path(string=w612) -> (path=w611:path)
            n279 = String To Path(string=w602) -> (path=w603:path)
            n280 = call <vilib>:"Check if File or Folder Exists.vi"("path"=w611) -> ("file or folder exists?"=→"上段":bool)  [unwired: 8 in, 2 out]
            n281 = call <vilib>:"Check if File or Folder Exists.vi"("path"=w603) -> ("file or folder exists?"=→"下段":bool)  [unwired: 8 in, 2 out]
            n282 = Close File(refnum=w607, error in=w606) -> (error out=w608:errorcluster)  [unwired: 1 out]
            n283 = call <vilib>:"Simple Error Handler.vi"("error in (no error)"=w608) -> ()  [unwired: 4 in, 5 out]
          }
        }
        n284 = for {
          N: 15 -> [_]
          shift-right: [w584] -> w514
          shift-left: w520 -> [w589]
          i -> [w591]
          n285 = Multiply(x=2, y=w591) -> (x*y=w588:i32)
          n286 = Increment(x=w588) -> (x+1=w587:i32)
          n287 = Index Array(array=w589, index #1=w588, index #2=w587) -> (element #1=w586:u16, element #2=w585:u16)
          n288 = Replace Array Subset(array=w589, new element #1=w585, index #1=w588, new element #2=w586, index #2=w587) -> (w584:u16[])
        }
        n289 = case shown="True" "更新物理参数" {
          tunnel: w524 -> [w593 w599]
          tunnel: w523 -> [w592 w598]
          tunnel: [w593 w597] -> w506
          tunnel: [w592 w596] -> w507
          tunnel: w514 -> [_ w594]
          frame False {
          }
          frame True {
            n290 = call-poly "MB Ethernet Master Query (poly).vi"("TCP Connection Refnum in"=w599, "Starting Address"=u16 194, "Registers"=w594, "error in"=w598) -> ("TCP Connection Refnum (dup)"=w597:refnum<k5>, "error out"=w596:errorcluster)  [unwired: 2 in, 12 out]
          }
        }
        n291 = case shown="True" "校准时间" {
          tunnel: w506 -> [w569 w575]
          tunnel: w507 -> [w568 w574]
          tunnel: [w569 w573] -> w505
          tunnel: [w568 w572] -> w504
          tunnel: w502 -> [_ w570]
          frame False {
          }
          frame True {
            n292 = call-poly "MB Ethernet Master Query (poly).vi"("TCP Connection Refnum in"=w575, "Starting Address"=u16 65436, "Registers"=w570, "error in"=w574) -> ("TCP Connection Refnum (dup)"=w573:refnum<k5>, "error out"=w572:errorcluster)  [unwired: 2 in, 12 out]
          }
        }
        n293 = flat-sequence {
          tunnel: w537 -> [w701]
          tunnel: w564 -> [w704]
          tunnel: [w701] -> w536
          frame #0 {
            n294 = Get Date/Time In Seconds() -> (seconds since 1Jan1904=w705:timestamp)
            n295 = Subtract(x=w705, y=w704) -> (x-y=w702:dbl)
            "电脑历时" <- w702
            n296 = Subtract(x=w702, y=w701) -> (x-y=→"累计时差":dbl)
            "程序历时" <- w701
          }
        }
        n297 = call-poly "MB Ethernet Master Query (poly).vi"("TCP Connection Refnum in"=w505, "Starting Address"=u16 0, "Quantity"=u16 30 ("modbus寄存器数量"), "Timeout"=500, "error in"=w504) -> ("TCP Connection Refnum (dup)"=w531:refnum<k5>, "Input Registers"=w510:u16[], "error out"=w532:errorcluster)  [unwired: 12 out]
        n298 = for {
          N: 15 -> [_]
          shift-right: [w576] -> w509
          shift-left: w510 -> [w581]
          i -> [w583]
          n299 = Multiply(x=2, y=w583) -> (x*y=w580:i32)
          n300 = Increment(x=w580) -> (x+1=w579:i32)
          n301 = Index Array(array=w581, index #1=w580, index #2=w579) -> (element #1=w578:u16, element #2=w577:u16)
          n302 = Replace Array Subset(array=w581, new element #1=w577, index #1=w580, new element #2=w578, index #2=w579) -> (w576:u16[])
        }
        n303 = Type Cast(type=w512, x=w509) -> (*(type *) &x=w547:sgl[])
        n304 = Array Subset(array=w547, index=0 ("索引"), length=3 ("长度")) -> (w553:sgl[])
        n305 = Array Subset(array=w547, index=3 ("索引"), length=8 ("长度")) -> (w550:sgl[])
        n306 = Array Subset(array=w547, index=11 ("索引"), length=2 ("长度")) -> (w546:sgl[])
        n307 = To Double Precision Float(number=w550) -> (double precision float=w556:dbl[])
        n308 = for {
          tunnel: w556 -> [w644] mode=indexing
          tunnel: [w643] -> w559 mode=indexing
          tunnel: w563 -> [w646]
          i -> [w645]
          n309 = Index Array(array=w646, index (row)=w645) -> (element=w647:dbl[])  [unwired: 1 in]
          n310 = call-poly <vilib>:"Polynomial Evaluation.vi"("P(x)"=w647, "a"=w644) -> ("P(a)"=w643:dbl)  [unwired: 1 out]
        }
        n311 = for {
          tunnel: w559 -> [w659] mode=indexing
          tunnel: [w658] -> w558 mode=indexing
          tunnel: w560 -> [w660] mode=indexing
          tunnel: w561 -> [w657] mode=indexing
          n312 = Equal?(x=w657, y=sgl 0.0) -> (x = y?=w654:bool)
          n313 = Equal?(x=w657, y=sgl 2.0) -> (x = y?=w653:bool)
          n314 = Or(x=w654, y=w653) -> (x .or. y?=w652:bool)
          n315 = Index Array(array=w660) -> (element #1=w651:sgl, element #2=w650:sgl, element #3=w649:sgl, element #4=w648:sgl)  [unwired: 4 in]
          n316 = case shown="True" w652 {
            tunnel: w659 -> [w672 w678]
            tunnel: [w671 w676] -> w658
            tunnel: w649 -> [w664 w681]
            tunnel: w648 -> [w663 w680]
            tunnel: w651 -> [w662 w674]
            tunnel: w650 -> [w661 w679]
            frame False {
              # "b"
              # "k"
              n317 = Subtract(x=w664, y=w663) -> (x-y=w669:sgl)
              n318 = Subtract(x=w662, y=w661) -> (x-y=w670:sgl)
              n319 = Divide(x=w670, y=w669) -> (x/y=w668:sgl)
              n320 = Multiply(x=w672, y=w668) -> (x*y=w666:dbl)
              n321 = Multiply(x=w668, y=w663) -> (x*y=w667:sgl)
              n322 = Subtract(x=w661, y=w667) -> (x-y=w665:sgl)
              n323 = Add(x=w666, y=w665) -> (x+y=w671:dbl)
            }
            frame True {
              # "b"
              # "k"
              n324 = Logarithm Base 10(1:w674) -> (0:w673:sgl)
              n325 = Logarithm Base 10(1:w679) -> (0:w675:sgl)
              n326 = Subtract(x=w681, y=w680) -> (x-y=w686:sgl)
              n327 = Subtract(x=w673, y=w675) -> (x-y=w687:sgl)
              n328 = Divide(x=w687, y=w686) -> (x/y=w685:sgl)
              n329 = Multiply(x=w678, y=w685) -> (x*y=w683:dbl)
              n330 = Multiply(x=w685, y=w680) -> (x*y=w684:sgl)
              n331 = Subtract(x=w675, y=w684) -> (x-y=w682:sgl)
              n332 = Add(x=w683, y=w682) -> (x+y=w677:dbl)
              n333 = Power Of 10(x=w677) -> (10^x=w676:dbl)
            }
          }
        }
        n334 = To Double Precision Float(number=w546) -> (double precision float=w545:dbl[])
        n335 = To Unsigned Long Integer(number=w553) -> (unsigned 32bit integer=w557:u32[])
        n336 = global read "GlobalVariable.vi" "电压输出"() -> (w528:sgl[])
        n337 = global read "GlobalVariable.vi" "V输出mbHR地址"() -> (w527:u16[])
        n338 = Index Array(array=w557) -> (element #1=→"脉冲1":u32, element #2=→"脉冲2":u32, element #3=→"脉冲3":u32)  [unwired: 3 in]
        n339 = Index Array(array=w559) -> (element #1=→"电压1":dbl, element #2=→"电压2":dbl, element #3=→"电压3":dbl, element #4=→"电压4":dbl, element #5=→"电压5":dbl, element #6=→"电压6":dbl, element #7=→"电压7":dbl, element #8=→"电压8":dbl)  [unwired: 8 in]
        n340 = Index Array(array=w558) -> (element #1=→"P2_1":dbl, element #2=→"P2_2":dbl, element #3=→"P2_3":dbl, element #4=→"P2_4":dbl, element #5=→"P2_5":dbl, element #6=→"P2_6":dbl, element #7=→"P2_7":dbl, element #8=→"P2_8":dbl)  [unwired: 8 in]
        n341 = flat-sequence {
          tunnel: w557 -> [w690]
          tunnel: w545 -> [w691]
          tunnel: w558 -> [w692]
          tunnel: [w692] -> w567
          tunnel: [w691] -> w566
          tunnel: [w690] -> w565
          tunnel: w567 -> [w698]
          tunnel: w566 -> [w697]
          tunnel: w565 -> [w696]
          frame #0 {
            n342 = global read "GlobalVariable.vi" "有无接收"() -> (w689:bool)
            n343 = case shown="True" w689 {
              frame False {
              }
              frame True {
                n344 = while {
                  stop <- w694 stop-if-true
                  n345 = global read "GlobalVariable.vi" "读完毕"() -> (w693:bool)
                  n346 = local read "退出"() -> (w695:bool)
                  n347 = Or(x=w693, y=w695) -> (x .or. y?=w694:bool)
                }
              }
            }
          }
          frame #1 {
            n348 = global write "GlobalVariable.vi" "计数率"(w696) -> ()
            n349 = global write "GlobalVariable.vi" "电压"(w698) -> ()
            n350 = global write "GlobalVariable.vi" "电流"(w697) -> ()
          }
          frame #2 {
            n351 = global write "GlobalVariable.vi" "写完毕"(TRUE ("写完毕")) -> ()
            n352 = global write "GlobalVariable.vi" "读完毕"(FALSE ("写完毕")) -> ()
          }
        }
        n353 = Index Array(array=w545) -> (element #1=→"电流 1":dbl, element #2=→"电流 2":dbl)  [unwired: 2 in]
        n354 = for {
          tunnel: w532 -> [w635]
          tunnel: w531 -> [w634]
          tunnel: [w633] -> w530
          tunnel: [w632] -> w529
          tunnel: w528 -> [w631] mode=indexing
          tunnel: w527 -> [w630] mode=indexing
          n355 = Type Cast(type=u16[] [] ("Input Registers"), x=w631) -> (*(type *) &x=w628:u16[])
          n356 = Index Array(array=w628) -> (element #1=w627:u16, element #2=w626:u16)  [unwired: 2 in]
          n357 = Build Array(w626, w627) -> (w625:u16[])
          n358 = call-poly "MB Ethernet Master Query (poly).vi"("TCP Connection Refnum in"=w634, "Starting Address"=w630, "Registers"=w625, "Timeout"=u32 500, "error in"=w635) -> ("TCP Connection Refnum (dup)"=w632:refnum<k5>, "error out"=w633:errorcluster)  [unwired: 1 in, 12 out]
        }
        n359 = global read "GlobalVariable.vi" "子VI退出"() -> (w562:bool)
        n360 = local read "退出"() -> (w534:bool)
        n361 = case shown="True" w562 {
          frame False {
          }
          frame True {
            w688 = FALSE ("值(信号)")
            n362 = property on="Home Square" class="Bool (strict)"("Val(Sgnl)"=w688) -> ()  [unwired: 2 in, 2 out]
            n363 = global write "GlobalVariable.vi" "子VI退出"(w688) -> ()
          }
        }
        n364 = Unbundle By Name(w530) -> ("status"=w533:bool)
        n365 = Or(x=w533, y=w534) -> (x .or. y?=w535:bool)
      }
      n366 = TCP Close Connection ("关闭TCP连接")(connection ID=w311, error in (no error)=w310) -> ()  [unwired: 3 out]
    }
  }
  n367 = Current VI's Path() -> (path=w13:path)
  n368 = Strip Path(path=w13) -> (stripped path=w12:path)  [unwired: 1 out]
  n369 = while {
    shift-right: [w727] -> _
    shift-left: w16 -> [w722]
    shift-right: [w726] -> _
    shift-left: "" ("ItemTag") -> [w713]
    shift-right: [TRUE ("首循环时显示Logo")] -> _
    shift-left: w15 -> [w706]
    tunnel: w12 -> [w723]
    stop <- w724 stop-if-true
    # "用于退出另一个循环"
    n370 = case shown="True" w706 {
      tunnel: ["logo.vi" ("ItemTag") w784] -> w712
      tunnel: [TRUE w776] -> w707
      frame False {
      }
      frame True {
        n371 = event shown="[0] Menu Selection (User)" {
          selector: _ -> [_ _ _ _ _ _]
          dyn-events: _ -> [_ _ _ _ _ _]
          timeout: _ -> [_ _ _ _ _ _]
          tunnel: [w795 "logo.vi" ("ItemTag") "打开数据文件夹.vi" ("ItemTag") "堆物理参数设置.vi" ("ItemTag") "多通道并行实测\\多通道并行实测.vi" ("ItemTag") "周期拟合倒时反应性.vi" ("ItemTag")] -> w780
          tunnel: [w794 "仪器设置:" ("ItemPath") "" ("ItemPath") "仪器设置:" ("x") "实时测量:" ("x") "数据处理:" ("x")] -> w781
          event Menu Selection (User) {
            n372 = event-data() -> ("ItemPath"=w794:string, "MenuRef"=w796:refnum<k9>, "ItemTag"=w795:string)  [unwired: 1 out]
            n373 = case shown="Default" w795 {
              tunnel: w795 -> [_ w797]
              tunnel: w796 -> [_ w798]
              frame "About" {
                n374 = call "About.vi"() -> ()  [unwired: 1 out]
              }
              frame Default {
                n375 = Get Menu Item Info(7:w797, 11:w798) -> ()  [unwired: 1 in, 7 out]
              }
            }
          }
          event "Home Square": Value Change {
            n376 = event-data() -> ()  [unwired: 2 out]
          }
          event "Open Square": Value Change {
            n377 = event-data() -> ()  [unwired: 2 out]
          }
          event "Physics Parameters Square": Value Change {
            n378 = event-data() -> ()  [unwired: 2 out]
          }
          event "Measure Square": Value Change {
            n379 = event-data() -> ()  [unwired: 2 out]
            n380 = global write "GlobalVariable.vi" "有无接收"(FALSE ("有无接收")) -> ()
          }
          event "Calculate Square": Value Change {
            n381 = event-data() -> ()  [unwired: 2 out]
          }
        }
        n382 = flat-sequence {
          tunnel: [w788] -> w786
          tunnel: w780 -> [w787]
          tunnel: [w787] -> w785
          frame #0 {
            n383 = global read "GlobalVariable.vi" "有无接收"() -> (w788:bool)
          }
        }
        n384 = Search/Split String ("搜索/拆分字符串")(string=w781, search string/char (-)=":" ("搜索字符串/字符(-)")) -> (substring before match=w778:string)  [unwired: 1 in, 2 out]
        n385 = Equal?(x="仪器设置", y=w778) -> (x = y?=w775:bool)
        n386 = Equal?(x=w778, y="实时测量" ("x")) -> (x = y?=w777:bool)
        n387 = Or(x=w775, y=w777) -> (x .or. y?=w776:bool)
        n388 = case shown="True" w786 {
          tunnel: w785 -> [w789 w791]
          tunnel: [w789 w791] -> w784
          tunnel: w776 -> [_ w790]
          frame False {
          }
          frame True {
            n389 = flat-sequence {
              tunnel: w790 -> [w792]
              frame #0 {
                n390 = global write "GlobalVariable.vi" "返回LOGO"(w792) -> ()
              }
              frame #1 {
                n391 = while {
                  stop <- w793 continue-if-true
                  n392 = global read "GlobalVariable.vi" "返回LOGO"() -> (w793:bool)
                }
              }
            }
          }
        }
      }
    }
    n393 = Equal?(x=w712, y="MainExit") -> (x = y?=w717:bool)
    n394 = Not(x=w717) -> (.not. x?=w720:bool)
    n395 = local read "退出"() -> (w719:bool)
    n396 = Not Equal?(x=w713, y=w712) -> (x != y?=w714:bool)
    n397 = Or(x=w717, y=w719) -> (x .or. y?=w724:bool)
    n398 = And(x=w707, y=w714) -> (x .and. y?=w709:bool)
    n399 = local write "退出"(w724) -> ()
    n400 = And(x=w709, y=w720) -> (x .and. y?=w711:bool)
    n401 = Or(x=w709, y=w717) -> (x .or. y?=w716:bool)
    n402 = case shown="True" w716 {
      tunnel: w722 -> [w728 w731]
      tunnel: [w728 refnum<vi> refnum ("VI Ref")] -> w715
      frame False {
      }
      frame True {
        n403 = invoke class="VI" method="Abort VI"(reference=w731) -> (reference out=w732:refnum<vi>, error out=w733:errorcluster)  [unwired: 2 in, 1 out]
        n404 = Close Reference "关闭引用"(reference=w732, error in (no error)=w733) -> (error out=w729:errorcluster)
        n405 = invoke on="VI_Display" class="SubPnl" method="Remove VI"(error in=w729) -> ()  [unwired: 2 in, 3 out]
      }
    }
    n406 = Not(x=w706) -> (.not. x?=w708:bool)
    n407 = Or(x=w708, y=w711) -> (x .or. y?=w710:bool)
    n408 = case shown="True" w710 {
      tunnel: w715 -> [w739 _]
      tunnel: [w739 w762] -> w727
      tunnel: w712 -> [w735 w758]
      tunnel: [w736 w761] -> w726
      tunnel: w723 -> [w734 w760]
      tunnel: w713 -> [w737 _]
      tunnel: w707 -> [w738 _]
      frame False {
        n409 = case shown="True" w738 {
          tunnel: w737 -> [w754 _]
          tunnel: [w754 w755] -> w736
          tunnel: w735 -> [w743 w755]
          tunnel: w734 -> [w744 _]
          frame False {
            n410 = Build Path(base path=w744, name or relative path=w743) -> (appended path=w742:path)
            n411 = Open VI Reference(type specifier VI Refnum (for type only)=refnum<vi> refnum ("类型说明符VI引用句柄（仅用于类型）"), vi path=w742) -> (vi reference=w750:refnum<vi>, error out=w748:errorcluster)  [unwired: 4 in]
            n412 = invoke class="VI" method="FP.Open"(reference=w750, error in=w748, "Activate"=TRUE ("激活？"), "State"=T2."Standard" ("状态")) -> (reference out=w749:refnum<vi>, error out=w747:errorcluster)  [unwired: 1 in, 3 out]
            n413 = invoke class="VI" method="Run VI"(reference=w749, error in=w747, "Wait until done"=FALSE ("结束前等待"), "Auto Dispose Ref"=TRUE ("自动销毁引用")) -> (reference out=w741:refnum<vi>, error out=w740:errorcluster)  [unwired: 1 in, 3 out]
            n414 = Close Reference(reference=w741, error in (no error)=w740) -> ()  [unwired: 1 out]
          }
          frame True {
          }
        }
      }
      frame True {
        n415 = Equal?(x=w758, y="logo.vi") -> (x = y?=w757:bool)
        n416 = Build Path(base path=w760, name or relative path=w758) -> (appended path=w766:path)
        n417 = call "LoadAndRun.vi"("run?"=TRUE, "path"=w766) -> ("error out"=w763:errorcluster, "vi refnum out"=w764:refnum<vi>)  [unwired: 2 in]
        n418 = Not(x=w757) -> (.not. x?=w756:bool)
        n419 = case "条件结构" shown="False" w757 {
          tunnel: w758 -> [w770 w771]
          tunnel: w764 -> [w768 w772]
          tunnel: w763 -> [w769 _]
          tunnel: [w768 w772] -> w762
          tunnel: [w770 w771] -> w761
          frame False {
            n420 = invoke on="VI_Display" class="SubPnl" method="Insert VI"(error in=w769, "VI Ref"=w768) -> (error out=w767:errorcluster)  [unwired: 2 in, 3 out]
            n421 = call <vilib>:"Simple Error Handler.vi"("error in (no error)"=w767) -> ()  [unwired: 4 in, 5 out]
          }
          frame True {
          }
        }
        n422 = property on="VI_Display" class="SubPnl"("Visible"=w756) -> ()  [unwired: 2 in, 2 out]
      }
    }
    n423 = Wait (ms)(milliseconds to wait=50) -> ()  [unwired: 1 out]
  }
  n424 = while {
    stop <- w812 stop-if-true
    n425 = Get Date/Time In Seconds() -> (seconds since 1Jan1904=w816:timestamp)
    n426 = Get Date/Time String(date format (0)=enum16{"short", "long", "abbreviated"}."long" ("日期格式(0)"), seconds (now)=w816, want seconds? (F)=TRUE) -> (date string=→"日期":string, time string=→"时间":string)
    n427 = Wait (ms)(milliseconds to wait=u32 500) -> ()  [unwired: 1 out]
    n428 = local read "退出"() -> (w812:bool)
  }
  n429 = case shown="True" w4 {
    frame False {
      w817 = TRUE ("可见")
      n430 = property on="更新物理参数" class="Bool"("Visible"=w817) -> (error out=w818:errorcluster)  [unwired: 2 in, 1 out]
      n431 = property on="离线数据源" class="Bool"(error in=w818, "Visible"=w817) -> ()  [unwired: 1 in, 2 out]
    }
    frame True {
      n432 = invoke class="VI" method="FP.Close"() -> (reference out=w819:refnum<vi>, error out=w820:errorcluster)  [unwired: 3 in, 1 out]
      n433 = Close Reference(reference=w819, error in (no error)=w820) -> ()  [unwired: 1 out]
    }
  }
